vi "Ch_Active_Control_Client.vi"(2 "Match":string, 3 "Activate Channels?":bool, 4 "Control on":T7) -> (0 "Editted Channels":T1[](array[typedef]) {"Duty" format="%016b"; "D" format="%#_5g"; "C" format="%#_5g"; "B" format="%#_5g"; "A" format="%#_5g"}, 1 "No of Channels":i32)   [LabVIEW 2020]
uses:
  Sub VIs/Channel_State_Control.ctl
  Sub VIs/ADAM Controls/Ch_description_ADAM.ctl
  Sub VIs/ADAM Controls/Module_type_ADAM.ctl
  Sub VIs/ADAM Controls/Function_ADAM.ctl
  Sub VIs/ADAM Controls/Channel_State.ctl
  Sub VIs/ADAM Controls/Calib_type_ADAM.ctl
  Sub VIs/ADAM Controls/Address.ctl
  Anemometry/Anemometry Sub Vis/Globals/Preference_global.vi
panel:
  out "Iterations":i32
  in  "Ch Active Control":refnum<vi>
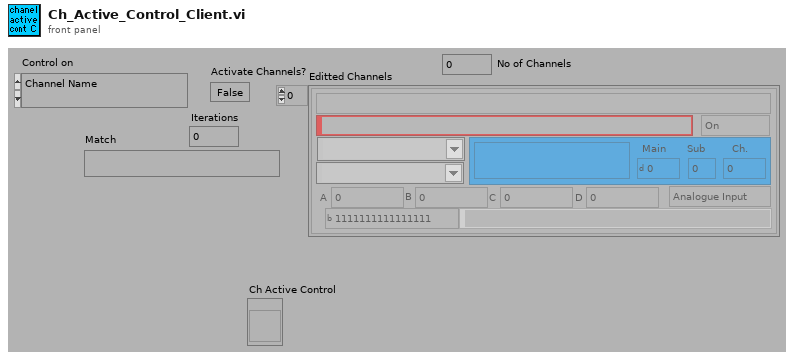
[diagram p1: front panel]
types:
  T1 = typedef "Ch_description_ADAM.ctl" = cluster{"Ch Name":string, "Type":T2, "Function":T3, "Ch State":T4, "Calibration type":T5, "A":dbl, "B":dbl, "C":dbl, "D":dbl, "Comments":string, "Address":T6, "String":string, "Duty":u16}
  T2 = typedef "Module_type_ADAM.ctl" = string
  T3 = typedef "Function_ADAM.ctl" = enum16{"Analogue Input", "Digital Input", "Event counter", "Event rate", "Analogue Output", "Digital Output", "Relay Output"}
  T4 = typedef "Channel_State.ctl" = enum16{"On", "Off", "Always On", "Always Off"}
  T5 = typedef "Calib_type_ADAM.ctl" = string
  T6 = typedef "Address.ctl" = cluster{"Main":i32, "Ch.":i32, "Sub":i32, "Port Name":string}
  T7 = typedef "Channel_State_Control.ctl" = enum16{"Channel Name", "Channel Name Starts with", "Main Address"}
  T8 = typedef "Server_Comms.ctl" = enum16{"Do Not Link To Server", "Server Link Healthy"}
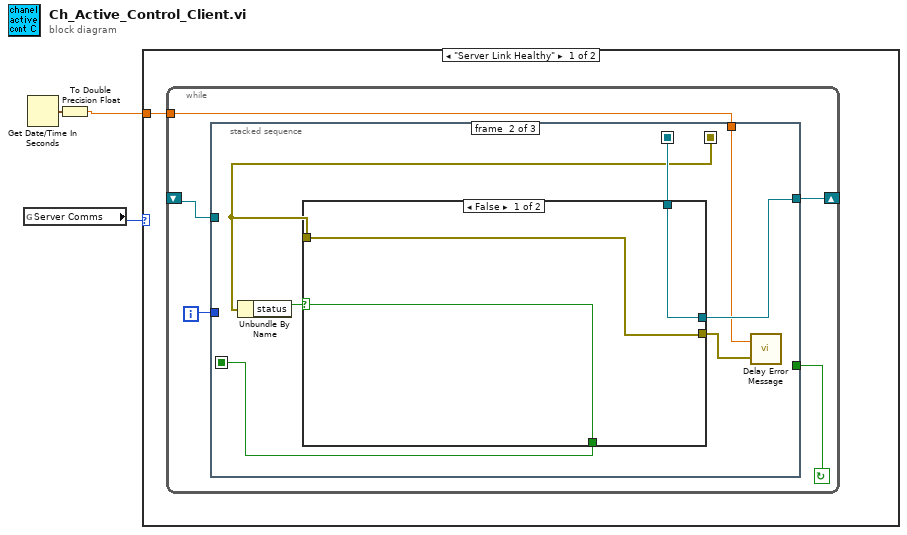
[diagram p0: block diagram]
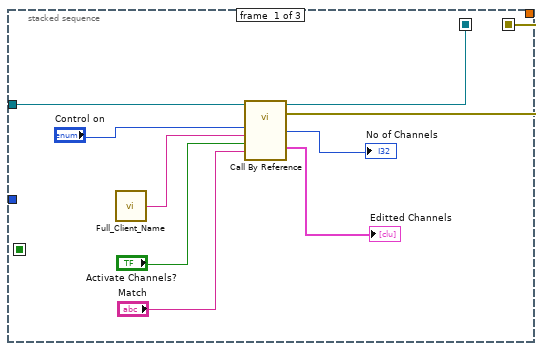
[diagram p2: hidden frame]
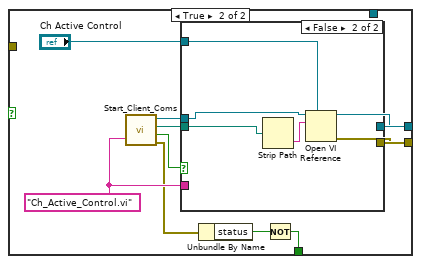
[diagram p3: hidden frame]
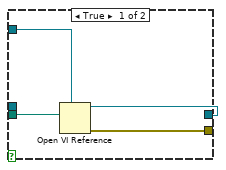
[diagram p4: hidden frame]
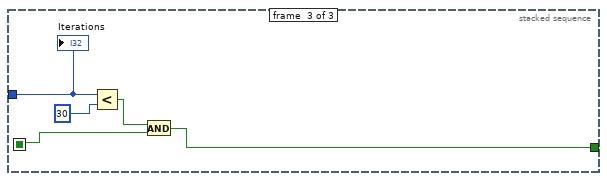
[diagram p5: hidden frame]
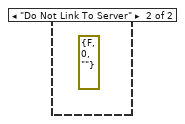
[diagram p6: hidden frame]
diagram:
  n1 = global read "Preference_global.vi" "Server Comms"() -> (w3:T8)
  n2 = Get Date/Time In Seconds() -> (seconds since 1Jan1904=w2:timestamp)
  n3 = To Double Precision Float(number=w2) -> (double precision float=w1:dbl)
  n4 = case shown="\"Server Link Healthy\"" w3 {
    tunnel: w1 -> [w4 _]
    frame "Server Link Healthy" {
      n5 = while {
        shift-left: _ -> [w9]
        shift-right: [w8] -> _
        tunnel: w4 -> [w5]
        i -> [w7]
        stop <- w6 continue-if-true
        n6 = stacked-sequence {
          seq-local: [w10 _ _] -> [_ w25 _]
          seq-local: [w18 _ _] -> [_ w23 _]
          seq-local: [_ w19 _] -> [_ _ w50]
          tunnel: w9 -> [w11 _ _]
          tunnel: [_ w22 _] -> w8
          tunnel: w7 -> [_ _ w51]
          tunnel: [_ _ w49] -> w6
          tunnel: w5 -> [_ w20 _]
          frame #0 {
            n7 = call "Full_Client_Name.vi"() -> ("Client Name"=w17:string)
            n8 = call-by-ref "?"(reference=w11, "Match"="Match", "Activate Channels?"="Activate Channels?", "Client Name"=w17, "Control on"="Control on") -> (reference out=w10:refnum<vi>, error out=w18:errorcluster, "Editted Channels"=→"Editted Channels":T1[], "No of Channels"=→"No of Channels":i32)  [unwired: 1 in]
          }
          frame #1 {
            n9 = Unbundle By Name(w23) -> ("status"=w24:bool)
            n10 = case shown="False" w24 {
              selector: w24 -> [w26 _]
              tunnel: w25 -> [w27 _]
              tunnel: [w28 w35] -> w21
              tunnel: w23 -> [w28 _]
              tunnel: [w27 w34] -> w22
              tunnel: [w26 w29] -> w19
              frame False {
              }
              frame True {
                w33 = "Ch_Active_Control.vi"
                n11 = call "Start_Client_Coms.vi"("VI name to run on server"=w33) -> ("LabVIEW application reference"=w38:refnum<vi>, "Checked VI name"=w36:path, "Local Call"=w37:bool, "Error cluster"=w30:errorcluster)  [unwired: 1 in]
                n12 = case shown="False" w37 {
                  tunnel: w36 -> [w42 w47]
                  tunnel: w38 -> [_ w46]
                  tunnel: [w41 w43] -> w35
                  tunnel: [w40 w44] -> w34
                  tunnel: w33 -> [_ _]
                  tunnel: "Ch Active Control" -> [w39 w45]
                  frame True {
                    n13 = Open VI Reference(type specifier VI Refnum (for type only)=w39, vi path=w42) -> (vi reference=w40:refnum<vi>, error out=w41:errorcluster)  [unwired: 1 in, 3 out]
                  }
                  frame False {
                    n14 = Strip Path(path=w47) -> (name=w48:string)  [unwired: 1 out]
                    n15 = Open VI Reference(type specifier VI Refnum (for type only)=w45, application reference (local)=w46, vi path=w48) -> (vi reference=w44:refnum<vi>, error out=w43:errorcluster)  [unwired: 1 in, 2 out]
                  }
                }
                n16 = Unbundle By Name(w30) -> ("status"=w31:bool)
                n17 = Not(x=w31) -> (.not. x?=w29:bool)
              }
            }
            n18 = call "Delay Error Message.vi"("error in (no error)"=w21, "Seconds since 1904"=w20) -> ()  [unwired: 2 in]
          }
          frame #2 {
            n19 = Less?(x=w51, y=30) -> (x < y?=w53:bool)
            n20 = And(x=w53, y=w50) -> (x .and. y?=w49:bool)
            "Iterations" <- w51
          }
        }
      }
    }
    frame "Do Not Link To Server" {
      (unwired) errorcluster {"status"=FALSE, "code"=0, "source"=""}
    }
  }
